vi "BL132 CAM0 Beampipe  MIN.vi"() -> ()   [LabVIEW 2019]
panel:
  out "BL132 COAX 2":T1(plugin-control)
  out "BL132 COAX":T1(plugin-control)
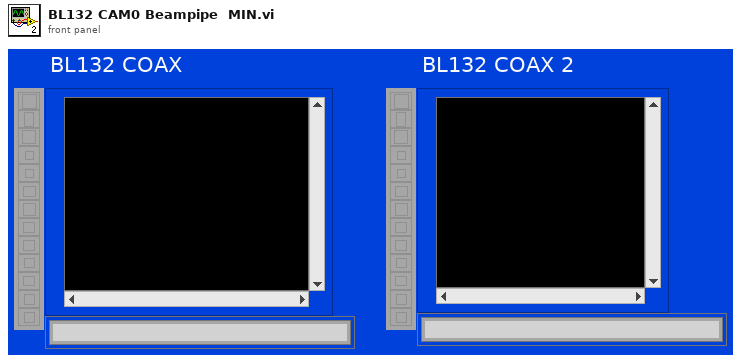
[diagram p1: front panel]
types:
  T1 = typedef "IMAQ Image.ctl" = refnum<image>
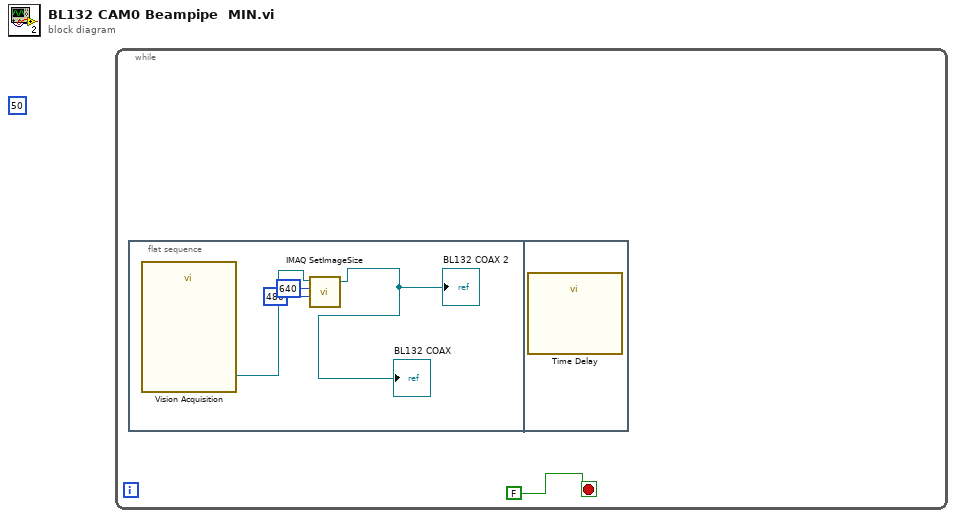
[diagram p0: block diagram]
diagram:
  (unwired) 50 ("Priority")
  n1 = while {
    stop <- FALSE stop-if-true
    n2 = flat-sequence {
      frame #0 {
        n3 = call "Vision Acquisition"() -> ("Image Out"=w5:T1)  [unwired: 26 in, 1 out]
        n4 = call "IMAQ SetImageSize"("Y Resolution"=480, "X Resolution"=640, "Image"=w5) -> ("Image Out"=→"BL132 COAX" →"BL132 COAX 2":T1)  [unwired: 2 in, 1 out]
      }
      frame #1 {
        n5 = call "Time Delay"() -> ()  [unwired: 11 in, 1 out]
      }
    }
  }
